vi "F_Active_B.vi"(8 "错误输入（无错误）":errorcluster, 10 "*.license文件路径":path, 11 "引用":refnum<k24>) -> (0 "错误输出":errorcluster, 2 "F_Active_B":bool, 3 "引用输出":refnum<k24>)   [LabVIEW 2013]
uses:
  AuthorizationToolClassLibrary.dll
panel:
  # "是否激活成功"
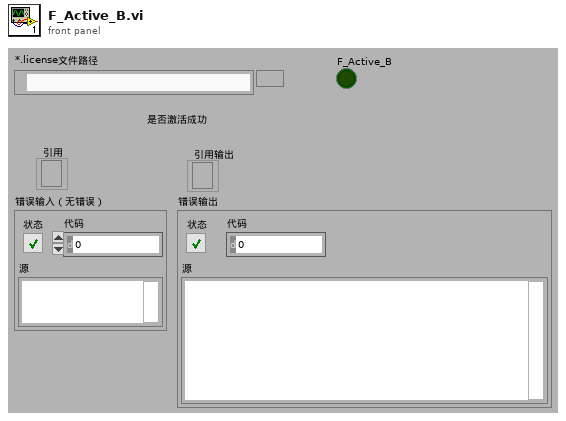
[diagram p1: front panel]
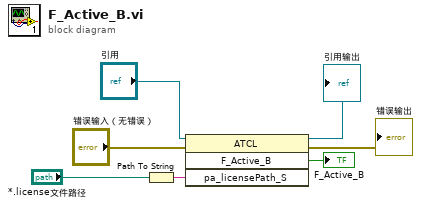
[diagram p0: block diagram]
diagram:
  n1 = Path To String(path="*.license文件路径") -> (string=w1:string)
  n2 = invoke class="ATCL" method="F_Active_B"(reference="引用", error in="错误输入（无错误）", "pa_licensePath_S"=w1) -> (reference out=→"引用输出":refnum<k24>, error out=→"错误输出":errorcluster, "F_Active_B"=→"F_Active_B":bool)  [unwired: 1 in, 1 out]
